vi "校正选择.vi"(10 "数值":dbl) -> ()   [LabVIEW 2012]
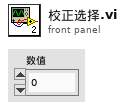
[diagram p1: front panel]
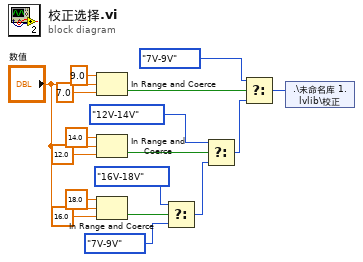
[diagram p0: block diagram]
diagram:
  n1 = In Range and Coerce(upper limit=9.0 ("上限"), x="数值", lower limit=7.0 ("下限")) -> (In Range?=w10:bool)  [unwired: 1 out]
  n2 = In Range and Coerce(upper limit=14.0 ("上限"), x="数值", lower limit=12.0 ("下限")) -> (In Range?=w8:bool)  [unwired: 1 out]
  n3 = In Range and Coerce(upper limit=18.0 ("上限"), x="数值", lower limit=16.0 ("下限")) -> (In Range?=w6:bool)  [unwired: 1 out]
  n4 = Select(t=enum16{"7V-9V", "12V-14V", "16V-18V"}."16V-18V" ("枚举"), s=w6, f=enum16{"7V-9V", "12V-14V", "16V-18V"}."7V-9V" ("枚举")) -> (s? t:f=w4:enum16{"7V-9V", "12V-14V", "16V-18V"})
  n5 = Select(t=enum16{"7V-9V", "12V-14V", "16V-18V"}."12V-14V" ("枚举"), s=w8, f=w4) -> (s? t:f=w3:enum16{"7V-9V", "12V-14V", "16V-18V"})
  n6 = Select(t=enum16{"7V-9V", "12V-14V", "16V-18V"}."7V-9V" ("枚举"), s=w10, f=w3) -> (s? t:f=w2:enum16{"7V-9V", "12V-14V", "16V-18V"})
  n7 = shared-variable ".\\未命名库 1.lvlib\\校正"(w2) -> ()  [unwired: 1 in, 1 out]
